vi "例4-31.vi"() -> ()   [LabVIEW 2019]
panel:
  out "强度图":i8[][](graph)
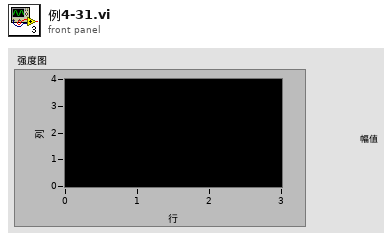
[diagram p1: front panel]
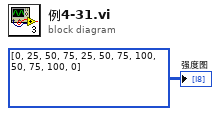
[diagram p0: block diagram]
diagram:
  "强度图" <- i8[][] [[0, 25, 50, 75], [25, 50, 75, 100], [50, 75, 100, 0]]
